vi "parse display.vi"(10 "result string":string="C.A.E.N. SY527 V3.18\rGROUP00\rCh_En is: On \rV0-SEL I0-SEL Crate 01\r\nChannel SVmax Rup Rdwn Trip TripEx PrOn PrOff Pon Pdwn Pswd On/Off Ch#\n*\nKLn_17 1000 100 100 010.0 -- 01 01 On Kill 1.00\nKLn_18 1980 100 100 010.0 -- 01 01 Off Kill 1.01\nKLn_19 2050 100 100 010.0 -- 01 01 Off Kill 1.02\nKLn_20 2004 100 100 010.0 -- 01 01 Off Kill 1.03\nKLn_21 2078 100 100 010.0 -- 01 01 Off Kill 1.04\nKLs_1 2142 100 100 010.0 -- 01 01 Off Kill 1.05\nKLs_2 2225 100 100 010.0 -- 01 01 Off Kill 1.06\nKLs_3 2162 100 100 010.0 -- 01 01 Off Kill 1.07\nKLs_4 2222 100 100 010.0 -- 01 01 Off Kill 1.08\nKLs_5 2182 100 100 010.0 -- 01 01 Off Kill 1.09\nKLs_6 2198 100 100 010.0 -- 01 01 Off Kill 1.10\nKLs_7 1775 100 100 010.0 -- 01 01 Off Kill 1.11\nKLs_8 1907 100 100 010.0 -- 01 01 Off Kill 1.12\nKLs_9 1897 100 100 010.0 -- 01 01 Off Kill 1.13\nKLs_10 1818 100 100 010.0 -- 01 01 Off Kill 1.14\nKLs_11 1936 100 100 010.0 -- 01 01 Off Kill 1.15\rA734 \rPage 1 \nKLn_17 \nQuit Edit Change Update Next Prev More Switch") -> (0 "error out":errorcluster, 1 "Tail":string, 2 "Table":string[][](table), 3 "Header":string, 4 "Subpage":i32, 5 "Column Headers":string[](array[string]), 6 "Page #":i32, 7 "Card Type":string)   [LabVIEW 2018]
uses:
  <vilib>/regexp/Match Regular Expression.xnode
panel:
  out "whole match":string
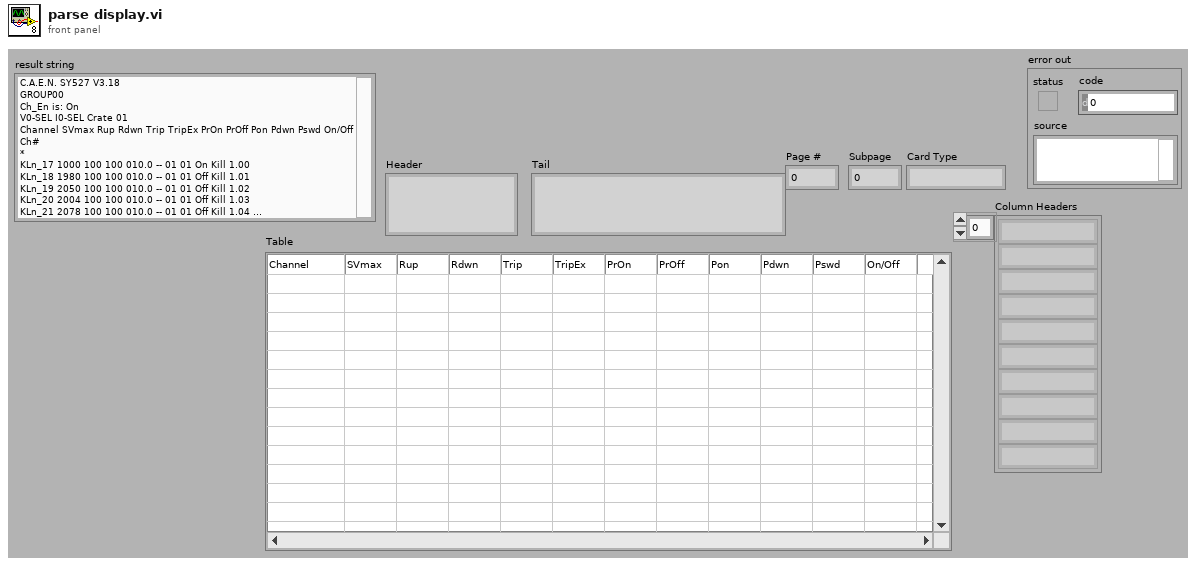
[diagram p1: front panel]
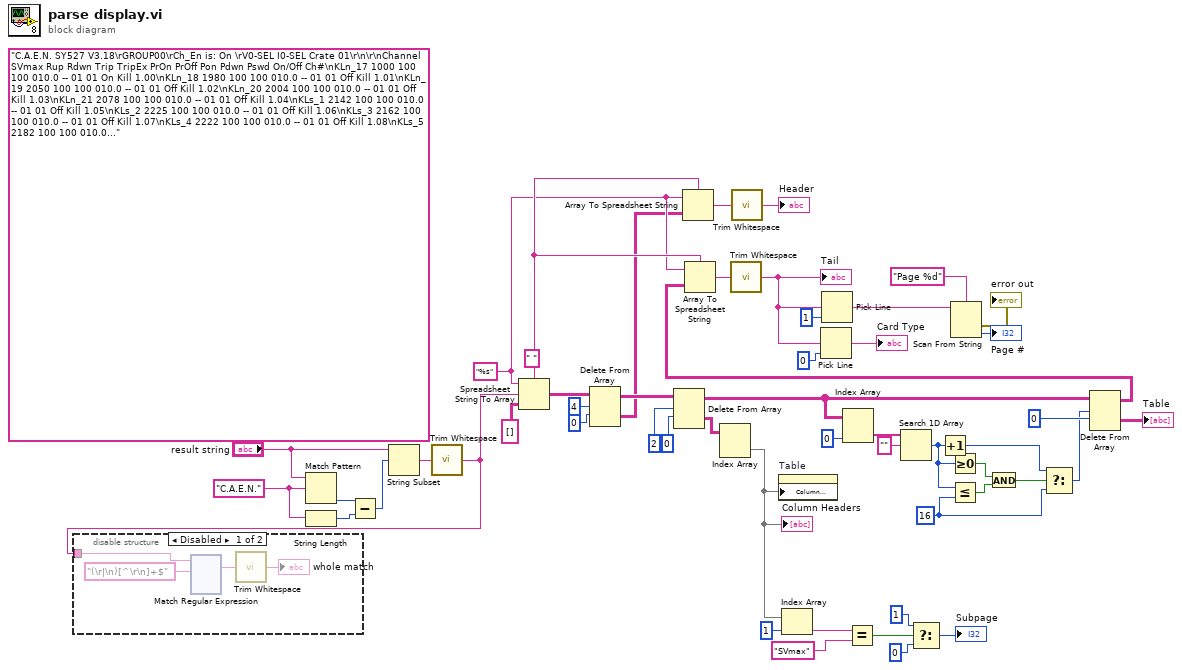
[diagram p0: block diagram]
diagram:
  w13 = "C.A.E.N." ("regular expression")
  w8 = 16 ("index (row)")
  (unwired) "C.A.E.N. SY527 V3.18\rGROUP00\rCh_En is: On \rV0-SEL I0-SEL Crate 01\r\n\r\nChannel SVmax Rup Rdwn Trip TripEx PrOn PrOff Pon Pdwn Pswd On/Off Ch#\nKLn_17 1000 100 100 010.0 -- 01 01 On Kill 1.00\nKLn_18 1980 100 100 010.0 -- 01 01 Off Kill 1.01\nKLn_19 2050 100 100 010.0 -- 01 01 Off Kill 1.02\nKLn_20 2004 100 100 010.0 -- 01 01 Off Kill 1.03\nKLn_21 2078 100 100 010.0 -- 01 01 Off Kill 1.04\nKLs_1 2142 100 100 010.0 -- 01 01 Off Kill 1.05\nKLs_2 2225 100 100 010.0 -- 01 01 Off Kill 1.06\nKLs_3 2162 100 100 010.0 -- 01 01 Off Kill 1.07\nKLs_4 2222 100 100 010.0 -- 01 01 Off Kill 1.08\nKLs_5 2182 100 100 010.0 -- 01 01 Off Kill 1.09\nKLs_6 2198 100 100 010.0 -- 01 01 Off Kill 1.10\nKLs_7 1775 100 100 010.0 -- 01 01 Off Kill 1.11\nKLs_8 1907 100 100 010.0 -- 01 01 Off Kill 1.12\nKLs_9 1897 100 100 010.0 -- 01 01 Off Kill 1.13\nKLs_10 1818 100 100 010.0 -- 01 01 Off Kill 1.14\nKLs_11 1936 100 100 010.0 -- 01 01 Off Kill 1.15\rA734 \rPage 1 \nKLn_17 \nQuit Edit Change Update Next Prev More Switch" ("result string")
  w48 = "%s" ("delimiter (Tab)")
  w49 = " " ("delimiter (Tab)")
  n1 = Match Pattern(string="result string", regular expression=w13) -> (offset past match=w12:i32)  [unwired: 1 in, 3 out]
  n2 = String Length(string=w13) -> (length=w11:i32)
  n3 = Subtract(x=w12, y=w11) -> (x-y=w10:i32)
  n4 = String Subset(string="result string", offset (0)=w10) -> (substring=w9:string)  [unwired: 1 in]
  n5 = call <vilib>:"Trim Whitespace.vi"("string"=w9) -> ("trimmed string"=w33:string)  [unwired: 1 in]
  n6 = disable-structure shown="Disabled" {
    disable-tunnel: w33 -> [w54 _]
    frame Disabled {
      n7 = xnode "Match Regular Expression"("input string"=w54, "regular expression"="(\r|\n)[^\r\n]+$") -> ("whole match"=w53:string)  [unwired: 4 in, 4 out]
      n8 = call <vilib>:"Trim Whitespace.vi"("string"=w53) -> ("trimmed string"=→"whole match":string)  [unwired: 1 in]
    }
    frame Enabled {
    }
  }
  n9 = Spreadsheet String To Array(delimiter (Tab)=w49, format string=w48, spreadsheet string=w33, array type (2D Dbl)=string[][] []) -> (array=w23:string[][])
  n10 = Delete From Array(array=w23, length=4 ("index"), index (row)=0 ("index")) -> (deleted portion=w22:string[][], array with subset deleted=w24:string[][])  [unwired: 1 in]
  n11 = Delete From Array(array=w24, length=2 ("disabled index (col)"), index (row)=0) -> (deleted portion=w2:string[][], array with subset deleted=w29:string[][])  [unwired: 1 in]
  n12 = Array To Spreadsheet String(delimiter (Tab)=w49, array=w22, 3:w48) -> (spreadsheet string=w16:string)
  n13 = Index Array(array=w2) -> (element=w1:string[])  [unwired: 2 in]
  "Column Headers" <- w1
  n14 = call <vilib>:"Trim Whitespace.vi"("string"=w16) -> ("trimmed string"=→"Header":string)  [unwired: 1 in]
  n15 = property on="Table" class="Tbl (strict)"("Column Headers[]"=w1) -> ()  [unwired: 2 in, 2 out]
  n16 = Index Array(array=w1, index=1) -> (element=w44:string)
  n17 = Index Array(array=w29, index (col)=0 ("disabled index (col)")) -> (element=w31:string[])  [unwired: 1 in]
  n18 = Equal?(x=w44, y="SVmax") -> (x = y?=w41:bool)
  n19 = Search 1D Array(1D array=w31, element="") -> (index of element=w7:i32)  [unwired: 1 in]
  n20 = Select(t=1 ("index"), s=w41, f=0 ("index")) -> (s? t:f=→"Subpage":i32)
  n21 = Increment(x=w7) -> (x+1=w20:i32)
  n22 = Greater Or Equal To 0?(x=w7) -> (x >= 0?=w6:bool)
  n23 = Less Or Equal?(x=w7, y=w8) -> (x <= y?=w5:bool)
  n24 = And(x=w6, y=w5) -> (x .and. y?=w4:bool)
  n25 = Select(t=w20, s=w4, f=w8) -> (s? t:f=w19:i32)
  n26 = Delete From Array(array=w29, length=w19, index (row)=0) -> (deleted portion=→"Table":string[][], array with subset deleted=w21:string[][])  [unwired: 1 in]
  n27 = Array To Spreadsheet String(delimiter (Tab)=w49, array=w21, 3:w48) -> (spreadsheet string=w18:string)
  n28 = call <vilib>:"Trim Whitespace.vi"("string"=w18) -> ("trimmed string"=w17:string)  [unwired: 1 in]
  "Tail" <- w17
  n29 = Pick Line(multi-line string=w17, line index=0) -> (output string=→"Card Type":string)  [unwired: 1 in]
  n30 = Pick Line(multi-line string=w17, line index=1) -> (output string=w37:string)  [unwired: 1 in]
  n31 = Scan From String(format string="Page %d", input string=w37) -> (error out=→"error out":errorcluster, output 1=→"Page #":i32)  [unwired: 3 in, 2 out]
